vi "Result.Create Txt Result State File.vi"(8 "error in (no error)":errorcluster, 9 "Path":path, 10 "Action":enum16{"Read", "Write"}(ring), 11 "ResultIn":T1={"State"=enum."Passing", "Code"=0, "Description"=""}) -> (0 "error out":errorcluster, 3 "ResultOut":T1={"State"=enum."Passing", "Code"=0, "Description"=""})   [LabVIEW 2018]
uses:
  <vilib>/KATE/SeqMgr/SeqMgr.Result Info.ctl
  <vilib>/KATE/SeqMgr/SeqMgr.Result State Enum.ctl
  Errors/Error.Error Code List.ctl
  <vilib>/KATE/SeqMgr/SeqMgr.lvlib
  <vilib>/KATE/Files/File Utils.lvlib
  <vilib>/KATE/Strings/String Utils.lvlib
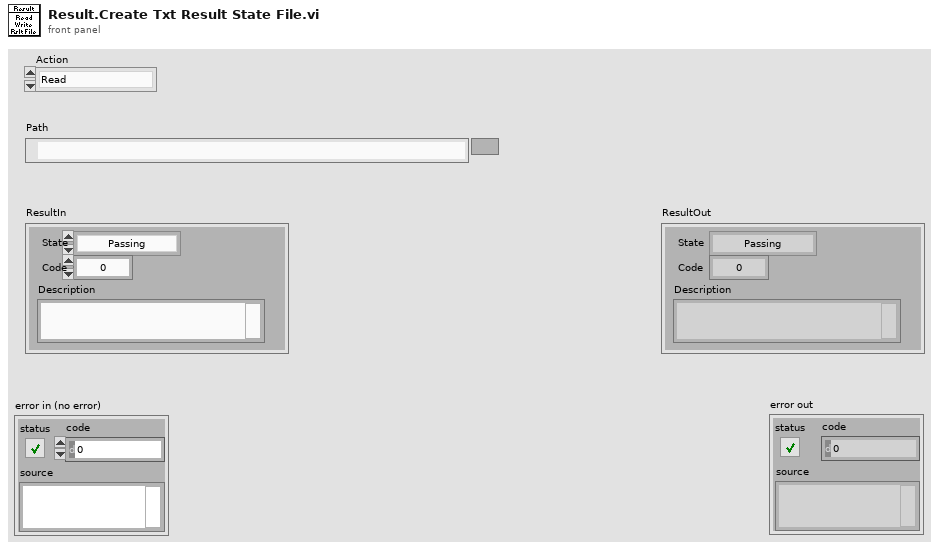
[diagram p1: front panel]
types:
  T1 = typedef "KATE_Lib.lvlib/SeqMgr.lvlib/SeqMgr.Result Info.ctl" = cluster{"State":T2, "Code":i32, "Description":string}
  T2 = typedef "KATE_Lib.lvlib/SeqMgr.lvlib/SeqMgr.Result State Enum.ctl" = enum16{"None", "Passing", "Failing", "PASS", "FAIL", "ABORT", "ERROR"}
  T3 = typedef "Error.Error Code List.ctl" = i32
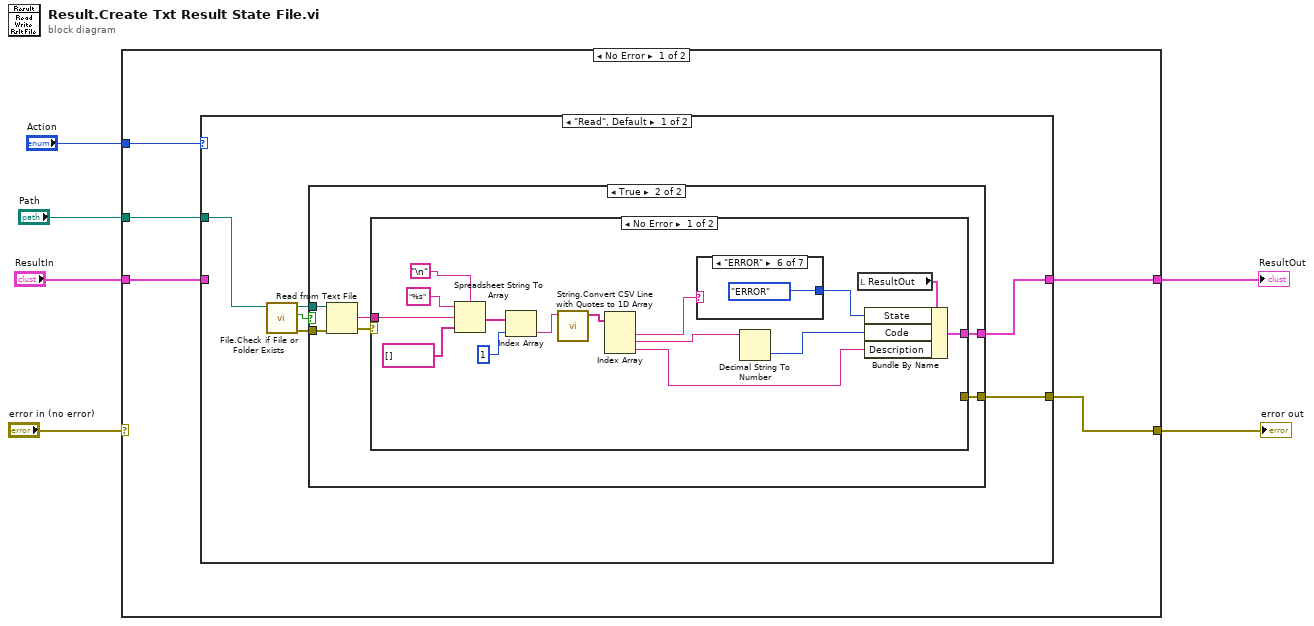
[diagram p0: block diagram]
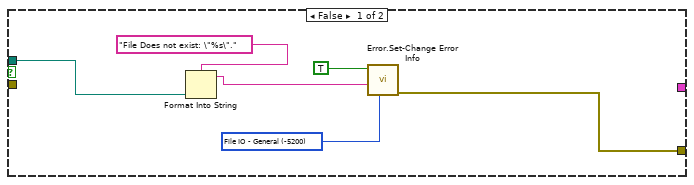
[diagram p2: hidden frame]
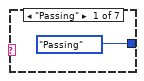
[diagram p3: hidden frame]
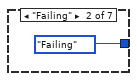
[diagram p4: hidden frame]
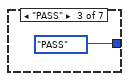
[diagram p5: hidden frame]
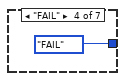
[diagram p6: hidden frame]
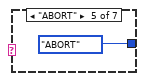
[diagram p7: hidden frame]
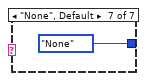
[diagram p8: hidden frame]
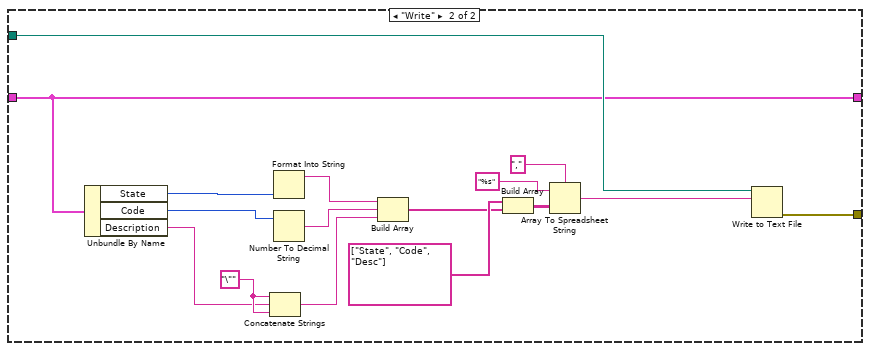
[diagram p10: hidden frame]
diagram:
  n1 = case shown="No Error" "error in (no error)" {
    selector: "error in (no error)" -> [_ w69]
    tunnel: [w11 w69] -> w6
    tunnel: "ResultIn" -> [w10 w70]
    tunnel: "Action" -> [w9 _]
    tunnel: "Path" -> [w8 _]
    tunnel: [w7 w70] -> w1
    frame No Error {
      n2 = case shown="\"Read\", Default" w9 {
        tunnel: [w16 w58] -> w11
        tunnel: w10 -> [_ w56]
        tunnel: w8 -> [w13 w57]
        tunnel: [w17 w56] -> w7
        frame "Read", Default {
          n3 = call <vilib>:"File.Check if File or Folder Exists.vi"("Path"=w13) -> ("error out"=w15:errorcluster, "Exists"=w12:bool, "Dup Path"=w14:path)  [unwired: 6 in, 2 out]
          n4 = case shown="True" w12 {
            tunnel: [_ w27] -> w17
            tunnel: [w19 w26] -> w16
            tunnel: w15 -> [_ w25]
            tunnel: w14 -> [w18 w24]
            frame False {
              w20 = T3 -5200 items=["No Error"=0, "Abort"=-2, "Misc"=-5000, "Fixture Error"=-5100, "File IO - General"=-5200, "FIle IO - Config Error"=-5201, "Instrument - General"=-5300, "Instrument - Serial Com"=-5301, "Instrument - Camera"=-5302, "Instrument - PS"=-5303, "Instrument - Oscilloscope"=-5304, "Instrument - Function Gen"=-5305, "Instrument - Load"=-5306, "Instrument - Meter"=-5307, "Instrument - Power Control"=-5308, "Instrument - Motion"=-5309, "Instrument - RF"=-5310, "System Exe"=-5400, "Image Processing"=-5500, "Communication"=-5600, "Script - Syntax Error"=-6000, "Script - Invalid Name or Param"=-6100, "Script - Timeout"=-6200, "Invalid Data"=-6300, "FW Update Error"=-6500] ("Std Code")
              n5 = Format Into String(format string="File Does not exist: \"%s\".", w18) -> (resulting string=w21:string)  [unwired: 2 in, 1 out]
              n6 = call "Error.Set-Change Error Info.vi"("Std Code"=w20, "Description"=w21, "Set Error"=TRUE) -> ("error out"=w19:errorcluster)  [unwired: 8 in]
            }
            frame True {
              n7 = Read from Text File(file (use dialog)=w24, error in=w25) -> (text=w28:string, error out=w29:errorcluster)  [unwired: 2 in, 2 out]
              n8 = case shown="No Error" w29 {
                selector: w29 -> [_ w52]
                tunnel: w28 -> [w44 _]
                tunnel: [w39 _] -> w27
                tunnel: [_ w52] -> w26
                frame No Error {
                  n9 = Spreadsheet String To Array(delimiter (Tab)="\n", format string="%s", spreadsheet string=w44, array type (2D Dbl)=string[] []) -> (array=w36:string[])
                  n10 = Index Array(array=w36, index=1) -> (element=w34:string)
                  n11 = call <vilib>:"String.Convert CSV Line with Quotes to 1D Array.vi"("CSV String"=w34) -> ("Array"=w33:string[])  [unwired: 9 in, 1 out]
                  n12 = Index Array(array=w33) -> (element #1=w32:string, element #2=w31:string, element #3=w30:string)  [unwired: 3 in]
                  n13 = case shown="\"ERROR\"" w32 {
                    tunnel: [SeqMgr.Result_State_Enum."Passing" ("State") SeqMgr.Result_State_Enum."Failing" ("State") SeqMgr.Result_State_Enum."PASS" ("State") SeqMgr.Result_State_Enum."FAIL" ("State") SeqMgr.Result_State_Enum."ABORT" ("State") SeqMgr.Result_State_Enum."ERROR" ("State") SeqMgr.Result_State_Enum."None" ("State")] -> w41
                    frame "Passing" {
                    }
                    frame "Failing" {
                    }
                    frame "PASS" {
                    }
                    frame "FAIL" {
                    }
                    frame "ABORT" {
                    }
                    frame "ERROR" {
                    }
                    frame "None", Default {
                    }
                  }
                  n14 = Decimal String To Number(string=w31) -> (number=w40:i32)  [unwired: 2 in, 1 out]
                  n15 = local read "ResultOut"() -> (w42:T1)
                  n16 = Bundle By Name(cluster=w42, "State"=w41, "Code"=w40, "Description"=w30) -> (w39:T1)
                }
                frame Error {
                }
              }
            }
          }
        }
        frame "Write" {
          w55 = "\""
          n17 = Unbundle By Name(w56) -> ("State"=w63:T2, "Code"=w68:i32, "Description"=w54:string)
          n18 = Concatenate Strings(w55, w54, w55) -> (w53:string)
          n19 = Format Into String(w63) -> (resulting string=w67:string)  [unwired: 3 in, 1 out]
          n20 = Number To Decimal String(number=w68) -> (decimal integer string=w66:string)  [unwired: 1 in]
          n21 = Build Array(w67, w66, w53) -> (w64:string[])
          n22 = Build Array(string[] ["State", "Code", "Desc"], w64) -> (w62:string[][])
          n23 = Array To Spreadsheet String(delimiter (Tab)=",", array=w62, 3:"%s" ("format string")) -> (spreadsheet string=w59:string)
          n24 = Write to Text File(file (use dialog)=w57, text=w59) -> (error out=w58:errorcluster)  [unwired: 2 in, 2 out]
        }
      }
    }
    frame Error {
    }
  }
  "ResultOut" <- w1
  "error out" <- w6
